vi "CAN Message Listing.vi"() -> ()   [LabVIEW 2014]
uses:
  Testing Code/NI-XNET Frame&Log - Converter.ctl
panel:
  out "size(s)":i32
  in  "stop":bool
  in  "group name":string="My Group"
  in  "channel name":string="My Channel"
  in  "File Path":path
  in  "Number of Frames to Read (-1:all)":i64=-1
  out "Frames Read":i32
  out "Frames":string[][](table)
  in  "Hexadecimal Display?":bool
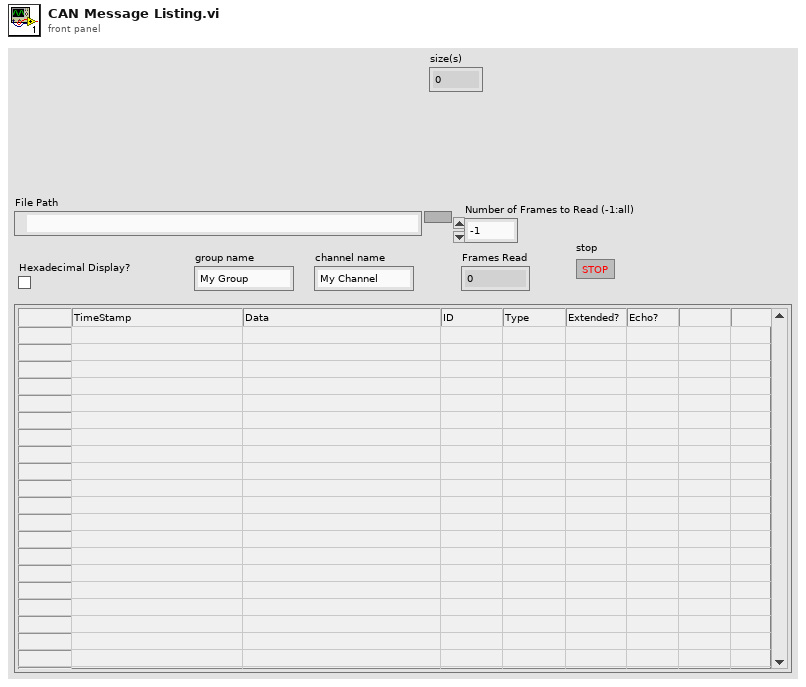
[diagram p1: front panel]
types:
  T1 = typedef "NI-XNET Frame&Log - Converter.ctl" = cluster{"endian swap?":bool, "partial":u8[], "index":i32}
  T2 = enum16{"big-endian, network order", "native, host order", "little-endian"}
  T3 = enum16{"open", "open or create", "create or replace", "create", "open (read-only)"}
  T4 = typedef "XNET Frame CAN.ctl" = cluster{"timestamp":timestamp, "payload":u8[], "identifier":u32, "type":T5, "extended?":bool, "echo?":bool}
  T5 = typedef "XNET Frame Type CAN.ctl" = u8
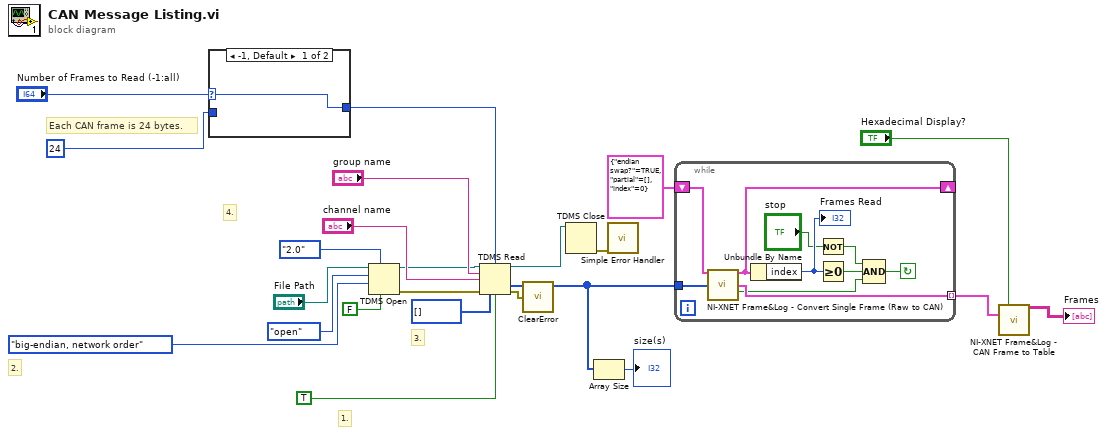
[diagram p0: block diagram]
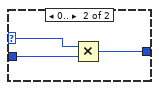
[diagram p2: hidden frame]
diagram:
  # "4."
  # "3."
  # "2."
  # "1."
  # "Each CAN frame is 24 bytes."
  n1 = case shown="-1, Default" "Number of Frames to Read (-1:all)" {
    selector: "Number of Frames to Read (-1:all)" -> [w24 w25]
    tunnel: i64 24 ("y") -> [_ w27]
    tunnel: [w24 w26] -> w16
    frame -1, Default {
    }
    frame 0.. {
      n2 = Multiply(x=w25, y=w27) -> (x*y=w26:i64)
    }
  }
  n3 = TDMS Open(6:FALSE ("disable buffering? (T)"), 7:enum16{"1.0", "2.0"}."2.0" ("file format version (2.0)"), 9:T2."big-endian, network order" ("byte order (2:little-endian)"), 10:T3."open" ("operation (0:open)"), 11:"File Path") -> (0:w6:errorcluster, 3:w7:refnum<k34>)  [unwired: 2 in]
  n4 = TDMS Read(0:w7, 2:w16, 5:"group name", 7:"channel name", 11:w6, 12:u8[] [] ("raw frames"), 13:TRUE ("return channels in file order? (F)")) -> (4:w19:refnum<k34>, 10:w2:u8[], 15:w13:errorcluster)  [unwired: 1 in, 3 out]
  n5 = call <vilib>:"ClearError.vi"("error in (no error)"=w13) -> ()  [unwired: 1 out]
  n6 = TDMS Close(11:w19) -> (0:w20:errorcluster)  [unwired: 1 in, 1 out]
  n7 = Array Size(array=w2) -> (size(s)=→"size(s)":i32)
  n8 = call <vilib>:"Simple Error Handler.vi"("error in (no error)"=w20) -> ()  [unwired: 1 in, 8 out]
  n9 = while {
    shift-right: [w35] -> _
    shift-left: T1 {"endian swap?"=TRUE, "partial"=[], "index"=0} ("converter  in") -> [w37]
    tunnel: w2 -> [w36]
    tunnel: [w33] -> w3 mode=indexing
    stop <- w30 continue-if-true
    n10 = call "NI-XNET Frame&Log - Convert Single Frame (Raw to CAN).vi"("converter  in"=w37, "raw frames"=w36) -> ("converter out"=w35:T1, "CAN frame"=w33:T4, "valid?"=w32:bool)  [unwired: 2 in, 9 out]
    n11 = Unbundle By Name(w35) -> ("index"=w34:i32)
    "Frames Read" <- w34
    n12 = Not(x="stop") -> (.not. x?=w28:bool)
    n13 = Greater Or Equal To 0?(x=w34) -> (x >= 0?=w31:bool)
    n14 = Compound Arithmetic op=AND(w28, w31, w32) -> (w30:bool)
  }
  n15 = call "NI-XNET Frame&Log - CAN Frame to Table.vi"("Hexadecimal?"="Hexadecimal Display?", "CAN Frames"=w3) -> ("Output Array"=→"Frames":string[][])  [unwired: 13 out]
